vi "global.vi"() -> ()   [LabVIEW 2019]
panel:
  out "BUTTON":bool
  out "TIMER":bool
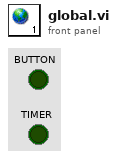
[diagram p1: front panel]
diagram:
